vi "FTW-Scheduler-Construct.vi"(5 "Initial Job Sequence":string, 11 "error in":errorcluster) -> (4 "FTW Job Scheduler":refnum<class "FTW-Scheduler.lvclass">, 15 "error out":errorcluster)   [LabVIEW 2015, in "FTW-Scheduler.lvclass"]
uses:
  FTW-Scheduler.lvclass
  FTW-Scheduler.lvclass/FTW-Scheduler.ctl
  lib/FTW-KernelFilepath.vi
panel:
  # "Inputs"
  # "Outputs"
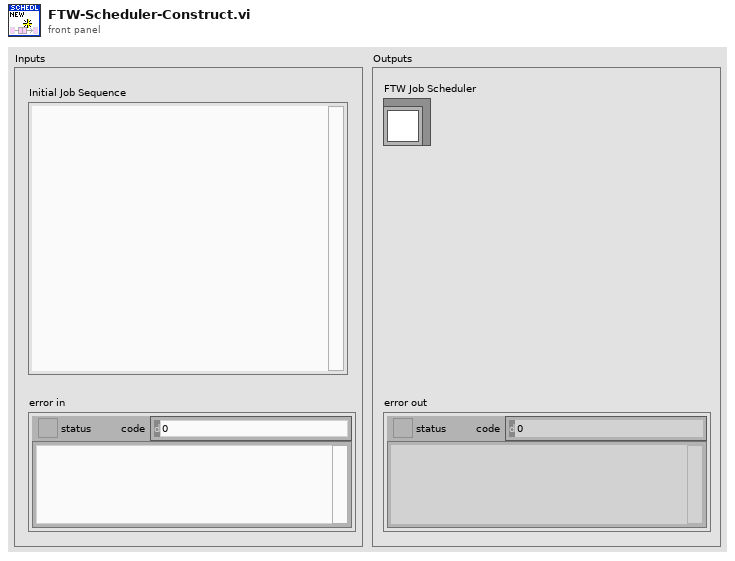
[diagram p1: front panel]
types:
  T1 = typedef "FTW-Type-JSON.ctl" = refnum<data-value>
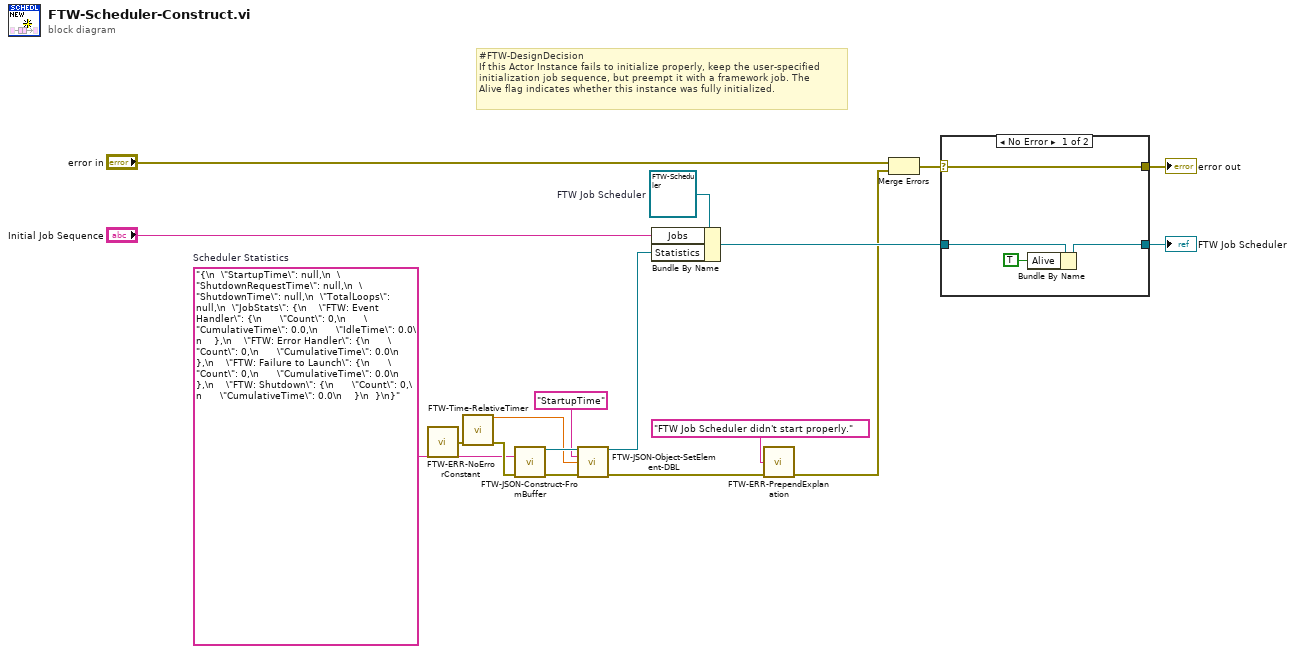
[diagram p0: block diagram]
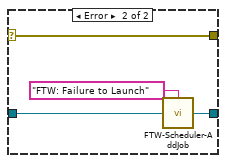
[diagram p2: hidden frame]
diagram:
  w13 = "{\n  \"StartupTime\": null,\n  \"ShutdownRequestTime\": null,\n  \"ShutdownTime\": null,\n  \"TotalLoops\": null,\n  \"JobStats\": {\n    \"FTW: Event Handler\": {\n      \"Count\": 0,\n      \"CumulativeTime\": 0.0,\n      \"IdleTime\": 0.0\n    },\n    \"FTW: Error Handler\": {\n      \"Count\": 0,\n      \"CumulativeTime\": 0.0\n    },\n    \"FTW: Failure to Launch\": {\n      \"Count\": 0,\n      \"CumulativeTime\": 0.0\n    },\n    \"FTW: Shutdown\": {\n      \"Count\": 0,\n      \"CumulativeTime\": 0.0\n    }\n  }\n}"  # Scheduler Statistics
  w18 = refnum<class "FTW-Scheduler.lvclass"> refnum  # FTW Job Scheduler
  # "#FTW-DesignDecision\nIf this Actor Instance fails to initialize properly, keep the user-specified\ninitialization job sequence, but preempt it with a framework job. The\nAlive flag indicates whether this instance was fully initialized."
  n1 = call "FTW-ERR-NoErrorConstant.vi"() -> ("no error"=w9:errorcluster)
  n2 = call "FTW-Time-RelativeTimer.vi"("error in"=w9) -> ("Current Timer Value"=w11:dbl, "error out"=w16:errorcluster)  [unwired: 12 in, 1 out]
  n3 = call "FTW-JSON-Construct-FromBuffer.vi"("JSON String (UTF-8)"=w13, "error in"=w16) -> ("JSON"=w15:T1, "error out"=w14:errorcluster)  [unwired: 12 in]
  n4 = call "FTW-JSON-Object-SetElement-DBL.vi"("JSON"=w15, "Key"="StartupTime", "Value"=w11, "error in"=w14) -> ("JSON out"=w10:T1, "error out"=w7:errorcluster)  [unwired: 10 in]
  n5 = Bundle By Name(cluster=w18, "Jobs"="Initial Job Sequence", "Statistics"=w10) -> (w8:refnum<class "FTW-Scheduler.lvclass">)
  n6 = call "FTW-ERR-PrependExplanation.vi"("Exception Information"="FTW Job Scheduler didn't start properly.", "error in"=w7) -> ("error out"=w4:errorcluster)  [unwired: 13 in]
  n7 = Merge Errors("error in", w4) -> (w3:errorcluster)
  n8 = case shown="No Error" w3 {
    selector: w3 -> [w21 w23]
    tunnel: w8 -> [w22 w26]
    tunnel: [w20 w24] -> w1
    tunnel: [w21 w23] -> w2
    frame No Error {
      n9 = Bundle By Name(cluster=w22, "Alive"=TRUE) -> (w20:refnum<class "FTW-Scheduler.lvclass">)
    }
    frame Error {
      n10 = call "FTW-Scheduler-AddJob.vi"("Add to Job Sequence"="FTW: Failure to Launch", "FTW Job Scheduler"=w26) -> ("FTW Job Scheduler out"=w24:refnum<class "FTW-Scheduler.lvclass">)  [unwired: 2 in]
    }
  }
  "FTW Job Scheduler" <- w1
  "error out" <- w2
